vi "Handle Group Subs.vi"(6 "Group":string, 9 "Timestamp":dbl, 10 "Data":dbl[](array[numeric]), 11 "Data Handlers":T1(c389)) -> ()   [LabVIEW 2020, in "Vecto.lvlib" / "RemoteDataService.lvclass"]
uses:
  RemoteDataService.lvclass
  SubscribedDataHandler/SubscribedDataHandler.lvclass
  Subscribed Data.ctl
  RemoteDataService.lvclass/RemoteDataService.ctl
  Vecto.lvlib
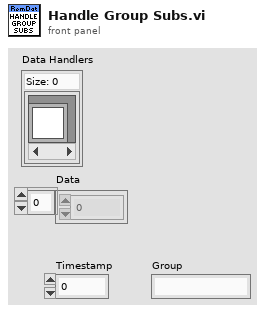
[diagram p1: front panel]
types:
  T1 = set{refnum<class "SubscribedDataHandler.lvclass">}
  T2 = typedef "Vecto.lvlib/Subscribed Data.ctl" = cluster{"Group":string, "Timestamp":dbl, "Data":dbl[], "Received Time":dbl}
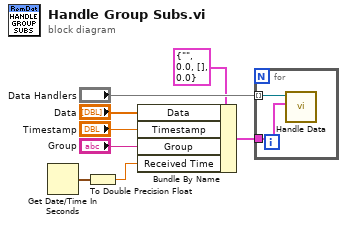
[diagram p0: block diagram]
diagram:
  n1 = Get Date/Time In Seconds() -> (seconds since 1Jan1904=w3:timestamp)
  n2 = To Double Precision Float(number=w3) -> (double precision float=w1:dbl)
  n3 = Bundle By Name(cluster=T2 {"Group"="", "Timestamp"=0.0, "Data"=[], "Received Time"=0.0} ("Subscribed Data"), "Data"="Data", "Timestamp"="Timestamp", "Group"="Group", "Received Time"=w1) -> (w4:T2)
  n4 = for {
    tunnel: "Data Handlers" -> [w10] mode=indexing
    tunnel: w4 -> [w9]
    n5 = call-dynamic "Handle Data.vi"("Data"=w9, "SubscribedDataHandler in"=w10) -> ()  [unwired: 9 in, 1 out]
  }
